vi "TCP Data Read.vi"(10 "Data":string, 11 "Head":string) -> (1 "Data Channel":i32, 2 "DataArray":dbl[](array[numeric]))   [LabVIEW 2020]
doc: "Reads an incoming package of data from a remote host via TCP/IP. This VI parses the package and extracts the data name and type as described in the meta data.\n\nFor the package to be parsed correctly, the meta data must be consistent in both the sender and the receiver. The data is packaged based on the existing meta data on the sender. Inconsistent meta data will result in inconsistent data parsing.\nUse the \"Read Meta\" and \"Write Meta\" VIs to ensure that both client and server have the same meta data.\n\nThe data is returned as a string. It is the responsibility of the user to cast it to the appropriate type before usage."
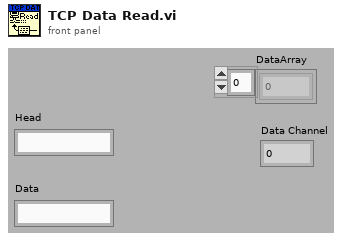
[diagram p1: front panel]
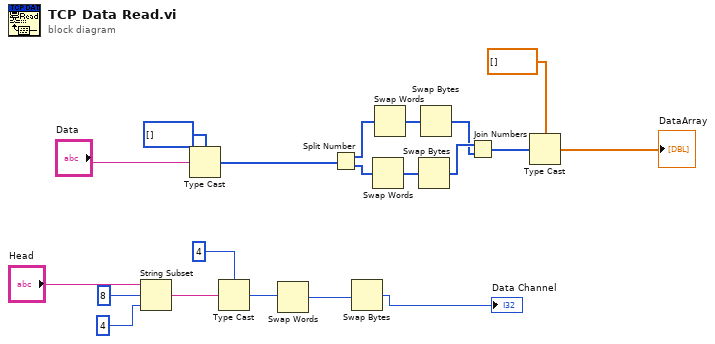
[diagram p0: block diagram]
diagram:
  n1 = String Subset(string="Head", offset (0)=8, length (rest)=4 ("length (rest)")) -> (substring=w9:string)
  n2 = Type Cast(type=i64[] [], x="Data") -> (*(type *) &x=w12:i64[])
  n3 = Type Cast(type=4 ("length (rest)"), x=w9) -> (*(type *) &x=w7:i32)
  n4 = Swap Words(1:w7) -> (0:w6:i32)
  n5 = Split Number(x=w12) -> (hi(x)=w14:u32[], lo(x)=w16:u32[])
  n6 = Swap Bytes(anything=w6) -> (byte swapped=→"Data Channel":i32)
  n7 = Swap Words(1:w16) -> (0:w15:u32[])
  n8 = Swap Words(1:w14) -> (0:w13:u32[])
  n9 = Swap Bytes(anything=w15) -> (byte swapped=w18:u32[])
  n10 = Swap Bytes(anything=w13) -> (byte swapped=w17:u32[])
  n11 = Join Numbers(hi=w18, lo=w17) -> ((hi.lo)=w19:u64[])
  n12 = Type Cast(type=dbl[] [], x=w19) -> (*(type *) &x=→"DataArray":dbl[])
